vi "Read Data Buffer.vi"(8 "error in (no error)":errorcluster, 9 "buffer (1:buffer 1)":u16(ring)=1 items=["Buffer 1"=1, "Buffer 2"=2], 11 "VISA resource name":refnum<visa-resource-name>) -> (0 "error out":errorcluster, 1 "data buffer":T1(array[cluster]) {"data" format="%.5e"}, 3 "VISA resource name out":refnum<visa-resource-name>)   [LabVIEW 2016, in "Agilent 4263X.lvlib"]
doc: "This VI reads back the current data buffer (one or two)."
uses:
  <instrlib>/Agilent 4263X/Agilent 4263X.lvlib
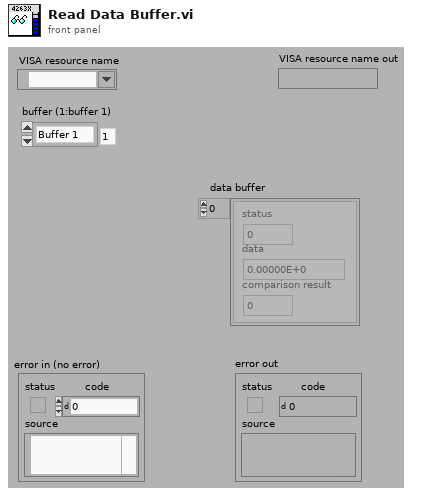
[diagram p1: front panel]
types:
  T1 = cluster{"status":u16, "data":dbl, "comparison result":u16}[]
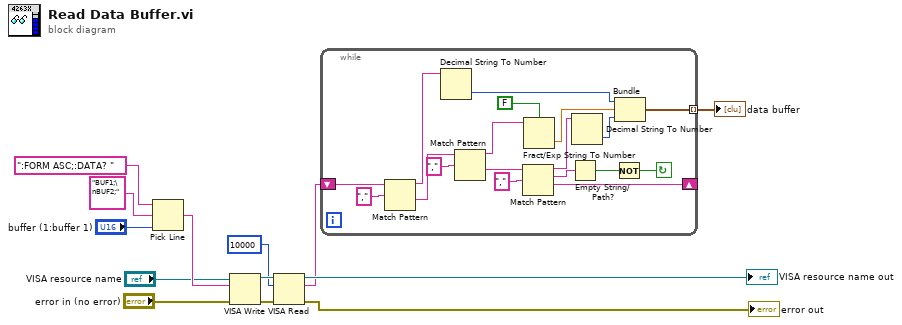
[diagram p0: block diagram]
diagram:
  n1 = Pick Line(string ("")=":FORM ASC;:DATA? ", multi-line string="BUF1;\nBUF2;", line index="buffer (1:buffer 1)") -> (output string=w13:string)
  n2 = VISA Write(VISA resource name="VISA resource name", write buffer=w13, error in (no error)="error in (no error)") -> (VISA resource name out=w11:refnum<visa-resource-name>, error out=w10:errorcluster)  [unwired: 1 out]
  n3 = VISA Read(VISA resource name=w11, byte count=10000, error in (no error)=w10) -> (VISA resource name out=→"VISA resource name out":refnum<visa-resource-name>, read buffer=w4:string, error out=→"error out":errorcluster)  [unwired: 1 out]
  n4 = while {
    tunnel: [w15] -> w3 mode=indexing
    shift-left: w4 -> [w22]
    shift-right: [w23] -> _
    stop <- w24 continue-if-true
    n5 = Match Pattern(string=w22, regular expression=",") -> (before substring=w21:string, after substring=w29:string)  [unwired: 1 in, 2 out]
    n6 = Decimal String To Number(string=w21) -> (number=w20:i32)  [unwired: 2 in, 1 out]
    n7 = Match Pattern(string=w29, regular expression=",") -> (before substring=w17:string, after substring=w28:string)  [unwired: 1 in, 2 out]
    n8 = Match Pattern(string=w28, regular expression=",") -> (before substring=w19:string, match substring=w26:string, after substring=w23:string)  [unwired: 1 in, 1 out]
    n9 = Fract/Exp String To Number(use system decimal point (T)=FALSE, string=w17) -> (number=w16:dbl)  [unwired: 2 in, 1 out]
    n10 = Empty String/Path?(string/path=w26) -> (empty?=w25:bool)
    n11 = Decimal String To Number(string=w19) -> (number=w18:i32)  [unwired: 2 in, 1 out]
    n12 = Not(x=w25) -> (.not. x?=w24:bool)
    n13 = Bundle(w20, w16, w18) -> (w15:cluster{i32, dbl, i32})  [unwired: 1 in]
  }
  "data buffer" <- w3
